vi "StepWithAssertPacket.vi"(11 "SequenceNumber":u32) -> (3 "StepWithAssertPacket":string)   [LabVIEW 2009]
panel:
  out "FCP Packet":u32[](array[numeric])
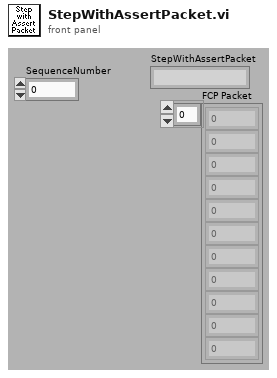
[diagram p1: front panel]
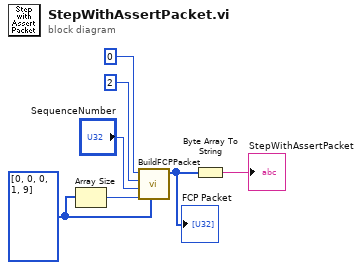
[diagram p0: block diagram]
diagram:
  w5 = u32[] [0, 0, 0, 1, 9] ("Data")
  n1 = Array Size(array=w5) -> (size(s)=w6:i32)
  n2 = call "BuildFCPPacket.vi"("Data"=w5, "Data Length (in Bytes)"=w6, "SequenceNumber"="SequenceNumber", "Channel"=u32 2, "Command"=u32 0) -> ("FCP Packet"=w2:u32[])  [unwired: 6 in]
  "FCP Packet" <- w2
  n3 = Byte Array To String(unsigned byte array=w2) -> (string=→"StepWithAssertPacket":string)
